vi "handle config error.vi"(8 "error in":errorcluster, 10 "return":i32, 11 "lvlibretls configurable context in":refnum<class "lvlibretls configurable context.lvclass">) -> (0 "error out":errorcluster)   [LabVIEW 2016, in "lvlibretls configurable context.lvclass"]
uses:
  lvlibretls configurable context.lvclass
  lvlibretls configurable context.lvclass/lvlibretls configurable context.ctl
  lv tls dll.lvlib
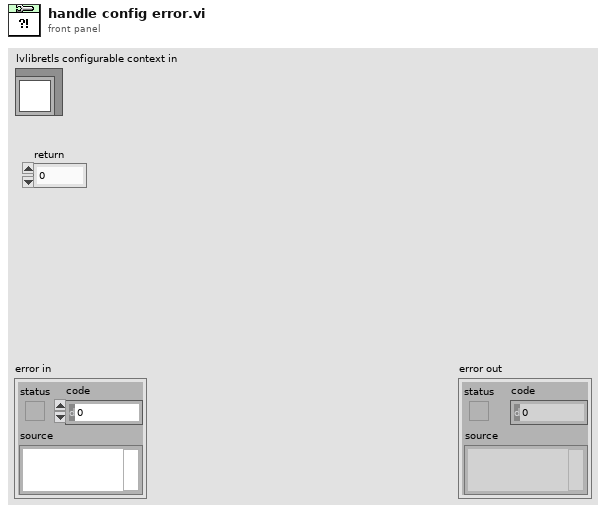
[diagram p1: front panel]
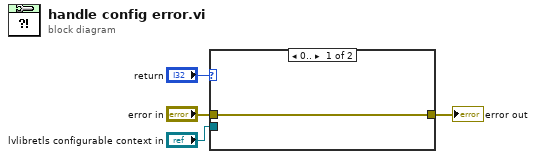
[diagram p0: block diagram]
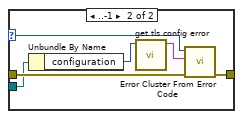
[diagram p2: hidden frame]
diagram:
  n1 = case shown="0.." "return" {
    selector: "return" -> [_ w7]
    tunnel: "error in" -> [w5 w11]
    tunnel: "lvlibretls configurable context in" -> [_ w10]
    tunnel: [w5 w8] -> w2
    frame 0.. {
    }
    frame ..-1 {
      n2 = Unbundle By Name(w10) -> ("configuration"=w9:u64)
      n3 = call "get tls config error.vi"("config"=w9) -> ("errString"=w6:string)  [unwired: 9 in, 1 out]
      n4 = call <vilib>:"Error Cluster From Error Code.vi"("error in (no error)"=w11, "error message (\"\")"=w6, "error code (0)"=w7) -> ("error out"=w8:errorcluster)  [unwired: 6 in]
    }
  }
  "error out" <- w2
